vi "DemoRS232.vi"() -> ()   [LabVIEW 2010]
uses:
  <vilib>/Instr/_visa.llb/VISA Configure Serial Port (Instr).vi
panel:
  out "read buffer 2":string
  out "status_1_OK":i32
  in  "CAN speed":u16(ring) items=["125 kBit", "500 kBit", "1000 kBit"]
  out "error out":errorcluster
  out "unsigned byte array":u8[](array[numeric])
  out "read buffer":string
  in  "Seria- Port":refnum<visa-resource-name>="COM5"
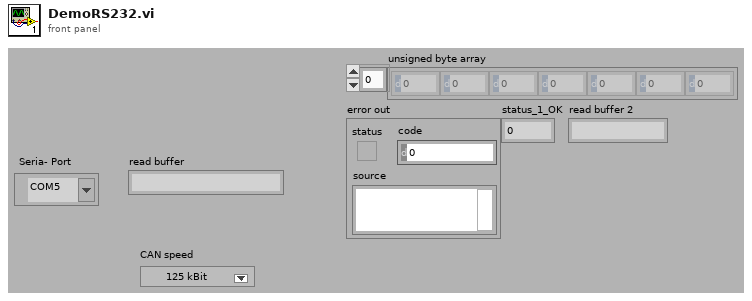
[diagram p1: front panel]
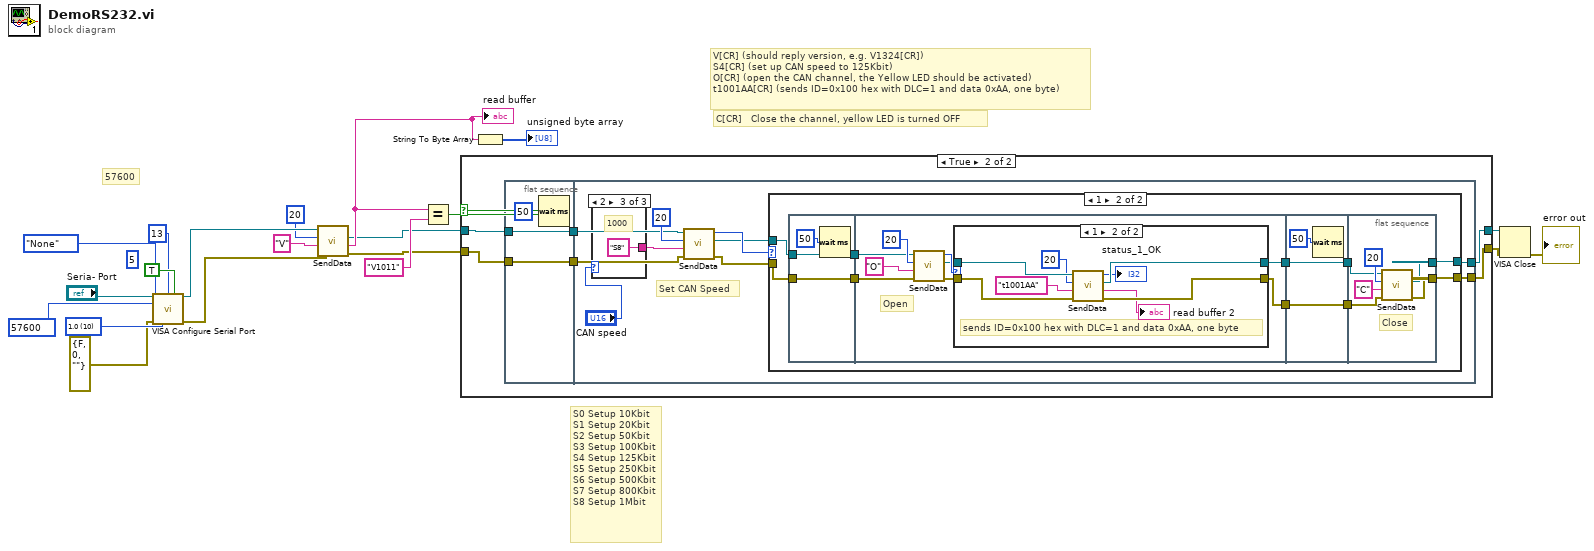
[diagram p0: block diagram]
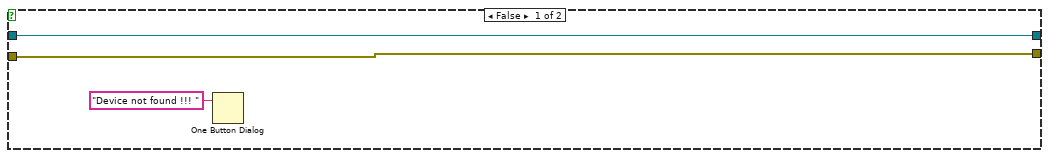
[diagram p2: hidden frame]
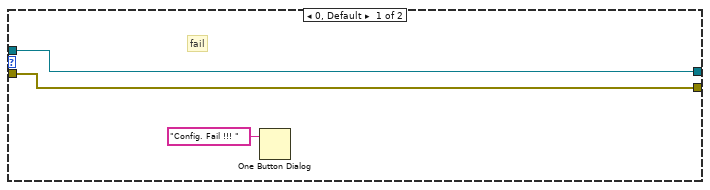
[diagram p3: hidden frame]
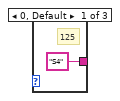
[diagram p5: hidden frame]
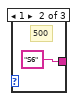
[diagram p6: hidden frame]
diagram:
  w17 = u32 57600 items=["4800"=4800, "9600"=9600, "19200"=19200, "38400"=38400, "57600"=57600, "115200"=115200] ("Baud rate")
  w16 = u16 10 items=["1.0"=10, "1.5"=15, "2.0"=20] ("stop bits")
  (unwired) u32 5 ("timeout (10sec)")
  # "C[CR]   Close the channel, yellow LED is turned OFF"
  # "S0 Setup 10Kbit\nS1 Setup 20Kbit\nS2 Setup 50Kbit\nS3 Setup 100Kbit\nS4 Setup 125Kbit\nS5 Setup 250Kbit\nS6 Setup 500Kbit\nS7 Setup 800Kbit\nS8 Setup 1Mbit"
  # "V[CR] (should reply version, e.g. V1324[CR])\nS4[CR] (set up CAN speed to 125Kbit)\nO[CR] (open the CAN channel, the Yellow LED should be activated)\nt1001AA[CR] (sends ID=0x100 hex with DLC=1 and data 0xAA, one byte)"
  # "57600"
  n1 = call-poly "VISA Configure Serial Port"("VISA resource name"="Seria- Port", "termination char\n(0xA = '\\n' = LF)"=u8 13 ("termination char\n(0xA = '\\n' = LF)"), "Enable Termination\nChar (T)"=TRUE ("Enable Termination\nChar (T)"), "baud rate (9600)"=w17, "parity (0:none)"=enum16{"None", "Odd", "Even", "Mark", "Space"}."None", "error in (no error)"=errorcluster {"status"=FALSE, "code"=0, "source"=""} ("error in"), "stop bits (10: 1 bit)"=w16) -> ("VISA resource name out"=w14:refnum<visa-resource-name>, "error out"=w13:errorcluster)  [unwired: 7 in]
  n2 = call "SendData.vi"("error out 2"=w13, "String"="V", "byte count"=u32 20, "VISA resource name out 2"=w14) -> ("error out"=w3:errorcluster, "read buffer"=w6:string, "VISA resource name out"=w4:refnum<visa-resource-name>)  [unwired: 1 out]
  "read buffer" <- w6
  n3 = Equal?(x=w6, y="V1011") -> (x = y?=w5:bool)
  n4 = case shown="True" w5 {
    tunnel: w4 -> [w23 w29]
    tunnel: w3 -> [w22 w28]
    tunnel: [w23 w25] -> w1
    tunnel: [w22 w24] -> w2
    frame False {
      n5 = One Button Dialog(message="Device not found !!! ") -> ()  [unwired: 1 in, 1 out]
    }
    frame True {
      n6 = flat-sequence {
        tunnel: w28 -> [w31]
        tunnel: w29 -> [w32]
        tunnel: [w32] -> w27
        tunnel: [w31] -> w26
        tunnel: w27 -> [w41]
        tunnel: w26 -> [w40]
        tunnel: [w33] -> w25
        tunnel: [w34] -> w24
        frame #0 {
          n7 = Wait (ms)(milliseconds to wait=u32 50) -> ()  [unwired: 1 out]
        }
        frame #1 {
          # "Set CAN Speed"
          n8 = case shown="2" "CAN speed" {
            tunnel: ["S4" "S6" "S8"] -> w38
            frame 0, Default {
              # "125"
            }
            frame 1 {
              # "500"
            }
            frame 2 {
              # "1000"
            }
          }
          n9 = call "SendData.vi"("error out 2"=w40, "String"=w38, "byte count"=u32 20, "VISA resource name out 2"=w41) -> ("error out"=w35:errorcluster, "VISA resource name out"=w36:refnum<visa-resource-name>, "status_1_OK"=w37:i32)  [unwired: 1 out]
          n10 = case shown="1" w37 {
            tunnel: w36 -> [w44 w54]
            tunnel: w35 -> [w43 w55]
            tunnel: [w44 w51] -> w33
            tunnel: [w43 w50] -> w34
            frame 0, Default {
              # "fail"
              n11 = One Button Dialog(message="Config. Fail !!! ") -> ()  [unwired: 1 in, 1 out]
            }
            frame 1 {
              n12 = flat-sequence {
                tunnel: w54 -> [w57]
                tunnel: w55 -> [w58]
                tunnel: [w58] -> w53
                tunnel: [w57] -> w52
                tunnel: w53 -> [w66]
                tunnel: w52 -> [w64]
                tunnel: [w60] -> w49
                tunnel: [w59] -> w47
                tunnel: w49 -> [w80]
                tunnel: [w80] -> w48
                tunnel: w47 -> [w79]
                tunnel: [w79] -> w46
                tunnel: [w82] -> w50
                tunnel: [w81] -> w51
                tunnel: w48 -> [w84]
                tunnel: w46 -> [w83]
                frame #0 {
                  n13 = Wait (ms)(milliseconds to wait=u32 50) -> ()  [unwired: 1 out]
                }
                frame #1 {
                  # "Open"
                  n14 = call "SendData.vi"("error out 2"=w66, "String"="O", "byte count"=u32 20, "VISA resource name out 2"=w64) -> ("error out"=w61:errorcluster, "VISA resource name out"=w62:refnum<visa-resource-name>, "status_1_OK"=w63:i32)  [unwired: 1 out]
                  n15 = case shown="1" w63 {
                    tunnel: w62 -> [w69 w76]
                    tunnel: [w69 w73] -> w60
                    tunnel: w61 -> [w68 w75]
                    tunnel: [w68 w72] -> w59
                    frame 0, Default {
                    }
                    frame 1 {
                      # "sends ID=0x100 hex with DLC=1 and data 0xAA, one byte"
                      n16 = call "SendData.vi"("error out 2"=w75, "String"="t1001AA", "byte count"=u32 20, "VISA resource name out 2"=w76) -> ("error out"=w72:errorcluster, "read buffer"=→"read buffer 2":string, "VISA resource name out"=w73:refnum<visa-resource-name>, "status_1_OK"=→"status_1_OK":i32)
                    }
                  }
                }
                frame #2 {
                  n17 = Wait (ms)(milliseconds to wait=u32 50) -> ()  [unwired: 1 out]
                }
                frame #3 {
                  # "Close"
                  n18 = call "SendData.vi"("error out 2"=w83, "String"="C", "byte count"=u32 20, "VISA resource name out 2"=w84) -> ("error out"=w82:errorcluster, "VISA resource name out"=w81:refnum<visa-resource-name>)  [unwired: 2 out]
                }
              }
            }
          }
        }
      }
    }
  }
  n19 = String To Byte Array(string=w6) -> (unsigned byte array=→"unsigned byte array":u8[])
  n20 = VISA Close(VISA resource name=w1, error in (no error)=w2) -> (error out=→"error out":errorcluster)
